vi "Write Period.vi"(8 "error in (no error)":errorcluster, 10 "Period":i16, 11 "Spk Cycle MSG in":refnum<class "Spk Cycle MSG.lvclass">) -> (0 "error out":errorcluster, 3 "Spk Cycle MSG out":refnum<class "Spk Cycle MSG.lvclass">)   [LabVIEW 2014, in "ePAS Library.lvlib" / "Spk Cycle MSG.lvclass"]
uses:
  Spk Cycle MSG.lvclass
  Spk Cycle MSG.lvclass/Spk Cycle MSG.ctl
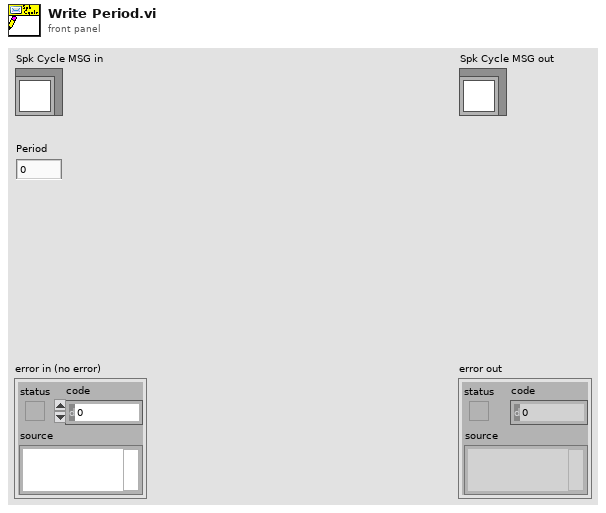
[diagram p1: front panel]
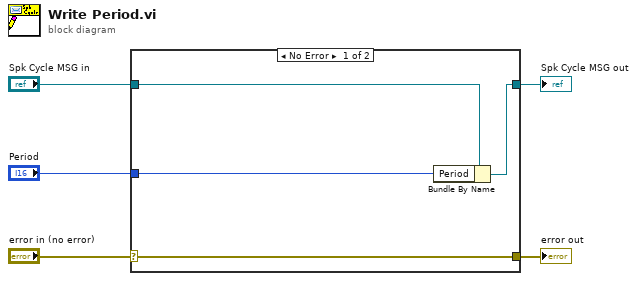
[diagram p0: block diagram]
diagram:
  n1 = case shown="No Error" "error in (no error)" {
    selector: "error in (no error)" -> [w9 w10]
    tunnel: [w9 w10] -> w4
    tunnel: [w7 w11] -> w2
    tunnel: "Spk Cycle MSG in" -> [w8 w11]
    tunnel: "Period" -> [w6 _]
    frame No Error {
      n2 = Bundle By Name(cluster=w8, "Period"=w6) -> (w7:refnum<class "Spk Cycle MSG.lvclass">)
    }
    frame Error {
    }
  }
  "error out" <- w4
  "Spk Cycle MSG out" <- w2
